vi "Finish.vi"   [LabVIEW 2013]
doc: "This VI is called just before exiting. It is expected to close I/O refnum, save collected data, etc."
uses:
  Systems/DriverStation/DriverStation.lvclass
  Systems/Compressor/Compressor.lvclass
  Systems/DriveMotors/DriveMotors.lvclass
  Systems/Blocker/Blocker.lvclass
  Systems/Catapult/Catapult.lvclass
  Systems/GrabberArms/GrabberArms.lvclass
  Systems/GrabberWheels/GrabberWheels.lvclass
  Systems/Shifter/Shifter.lvclass
  Robot Global Data.vi
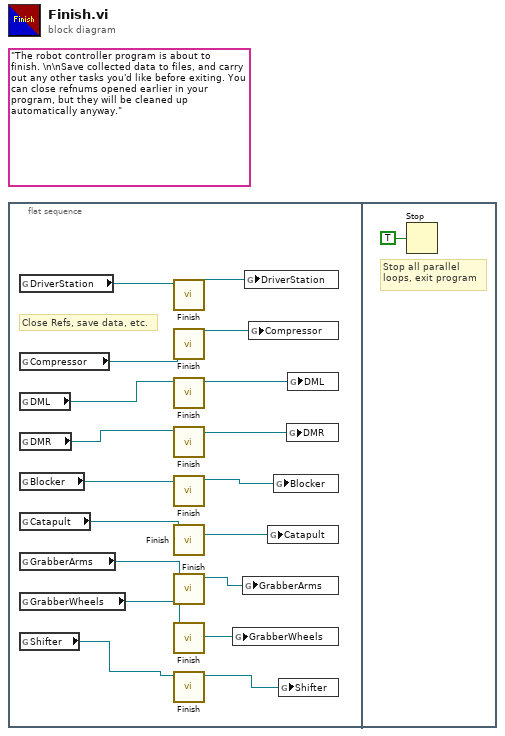
[diagram p0: block diagram]
diagram:
  (unwired) "The robot controller program is about to finish. \n\nSave collected data to files, and carry out any other tasks you'd like before exiting. You can close refnums opened earlier in your program, but they will be cleaned up automatically anyway."
  n1 = flat-sequence {
    frame #0 {
      # "Close Refs, save data, etc."
      n2 = global read "Robot Global Data.vi" "DriverStation"() -> (w18:refnum<class "DriverStation.lvclass">)
      n3 = global read "Robot Global Data.vi" "Compressor"() -> (w16:refnum<class "Compressor.lvclass">)
      n4 = global read "Robot Global Data.vi" "DML"() -> (w14:refnum<class "DriveMotors.lvclass">)
      n5 = global read "Robot Global Data.vi" "DMR"() -> (w13:refnum<class "DriveMotors.lvclass">)
      n6 = global read "Robot Global Data.vi" "Blocker"() -> (w8:refnum<class "Blocker.lvclass">)
      n7 = global read "Robot Global Data.vi" "Catapult"() -> (w12:refnum<class "Catapult.lvclass">)
      n8 = global read "Robot Global Data.vi" "GrabberArms"() -> (w11:refnum<class "GrabberArms.lvclass">)
      n9 = global read "Robot Global Data.vi" "GrabberWheels"() -> (w10:refnum<class "GrabberWheels.lvclass">)
      n10 = global read "Robot Global Data.vi" "Shifter"() -> (w9:refnum<class "Shifter.lvclass">)
      n11 = call-dynamic "Finish.vi"("DriverStation in"=w18) -> ("DriverStation out"=w17:refnum<class "DriverStation.lvclass">)  [unwired: 9 in, 1 out]
      n12 = call-dynamic "Finish.vi"("Compressor in"=w16) -> ("Compressor out"=w15:refnum<class "Compressor.lvclass">)  [unwired: 9 in, 1 out]
      n13 = call-dynamic "Finish.vi"("DriveMotors in"=w14) -> ("DriveMotors out"=w1:refnum<class "DriveMotors.lvclass">)  [unwired: 9 in, 1 out]
      n14 = call-dynamic "Finish.vi"("DriveMotors in"=w13) -> ("DriveMotors out"=w2:refnum<class "DriveMotors.lvclass">)  [unwired: 9 in, 1 out]
      n15 = call-dynamic "Finish.vi"("Blocker in"=w8) -> ("Blocker out"=w3:refnum<class "Blocker.lvclass">)  [unwired: 9 in, 1 out]
      n16 = call-dynamic "Finish.vi"("Catapult in"=w12) -> ("Catapult out"=w4:refnum<class "Catapult.lvclass">)  [unwired: 9 in, 1 out]
      n17 = call-dynamic "Finish.vi"("GrabberArms in"=w11) -> ("GrabberArms out"=w5:refnum<class "GrabberArms.lvclass">)  [unwired: 9 in, 1 out]
      n18 = call-dynamic "Finish.vi"("GrabberWheels in"=w10) -> ("GrabberWheels out"=w6:refnum<class "GrabberWheels.lvclass">)  [unwired: 9 in, 1 out]
      n19 = call-dynamic "Finish.vi"("Shifter in"=w9) -> ("Shifter out"=w7:refnum<class "Shifter.lvclass">)  [unwired: 9 in, 1 out]
      n20 = global write "Robot Global Data.vi" "GrabberWheels"(w6) -> ()
      n21 = global write "Robot Global Data.vi" "GrabberArms"(w5) -> ()
      n22 = global write "Robot Global Data.vi" "DriverStation"(w17) -> ()
      n23 = global write "Robot Global Data.vi" "Compressor"(w15) -> ()
      n24 = global write "Robot Global Data.vi" "Catapult"(w4) -> ()
      n25 = global write "Robot Global Data.vi" "Blocker"(w3) -> ()
      n26 = global write "Robot Global Data.vi" "Shifter"(w7) -> ()
      n27 = global write "Robot Global Data.vi" "DMR"(w2) -> ()
      n28 = global write "Robot Global Data.vi" "DML"(w1) -> ()
    }
    frame #1 {
      # "Stop all parallel\nloops, exit program"
      n29 = Stop(stop? (T)=TRUE ("Quit")) -> ()
    }
  }
